vi "Save_Info.vi"(8 "error in (no error)":errorcluster, 11 "Class in":refnum<class "Installer.lvclass">) -> (0 "error out":errorcluster, 3 "Class out":refnum<class "Installer.lvclass">)   [LabVIEW 2020, in "Installer.lvclass"]
uses:
  <vilib>/AppBuilder/IB_Classes/Installer/Installer.lvclass
  <vilib>/AppBuilder/IB_RW_Project/IB_RW_Project_PropBag_Action.ctl
  <resource>/Framework/Providers/Builds/Installer/CDK_sTypeDef_StorageReadWrite.ctl
  <vilib>/AppBuilder/IB_RW_Project/IB_RW_Project_Installer_Data.ctl
  <resource>/Framework/Providers/Builds/Installer/CDK_sTypeDef_Languages.ctl
  <resource>/Framework/Providers/Builds/Installer/CDK_sTypeDef_ProductVersion.ctl
panel:
  in  "Installer":T1={"author"="", "productName"="", "buildSpecName"="", "hide"=FALSE, "requireLVDevSys"=FALSE, "autoIncrement"=FALSE, "includeError"=FALSE, "readmeID"="", "buildLocation"=path "", "mediaSize"=0, "language"=9, "productVersion"={"Major"=1, "Minor"=0, "Update"=0}, "defaultDir"="", "web service itemIDs"=[], "installerName"=""} {"productVersion"."Update" step=1; "productVersion"."Minor" step=1; "productVersion"."Major" step=1; "language" items=["English"=9, "German"=7, "French"=12, "Japanese"=17, "Korean"=18, "Chinese (Simplified)"=2052]}
  # "."
  # "."
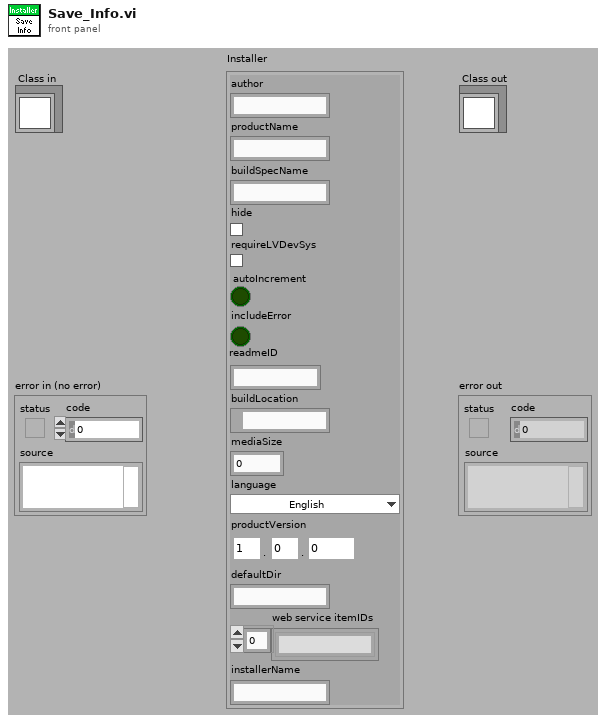
[diagram p1: front panel]
types:
  T1 = typedef "IB_RW_Project_Installer_Data.ctl" = cluster{"author":string, "productName":string, "buildSpecName":string, "hide":bool, "requireLVDevSys":bool, "autoIncrement":bool, "includeError":bool, "readmeID":string, "buildLocation":path, "mediaSize":u16, "language":T2, "productVersion":T3, "defaultDir":string, "web service itemIDs":string[], "installerName":string}
  T2 = typedef "CDK_sTypeDef_Languages.ctl" = u16
  T3 = typedef "CDK_sTypeDef_ProductVersion.ctl" = cluster{"Major":u8, "Minor":u8, "Update":u16}
  T4 = typedef "IB_RW_Project_PropBag_Action.ctl" = enum16{"read", "write", "clear", "readPrevious", "writePrevious", "clearPrevious"}
  T5 = typedef "CDK_sTypeDef_StorageReadWrite.ctl" = enum16{"Read", "Write", "Empty", "readPrevious"}
  T6 = typedef "ItemRef.ctl" = u64
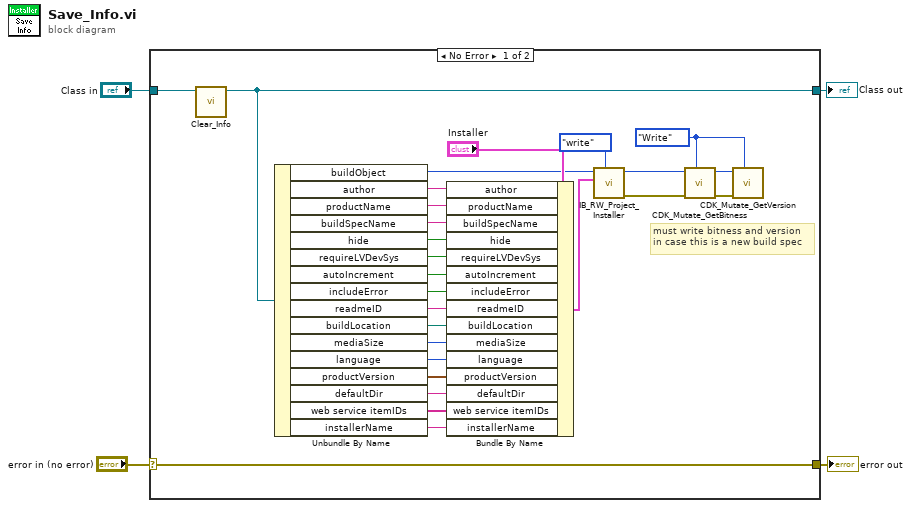
[diagram p0: block diagram]
diagram:
  n1 = case shown="No Error" "error in (no error)" {
    selector: "error in (no error)" -> [w29 w33]
    tunnel: [w29 w33] -> w3
    tunnel: [w13 w32] -> w1
    tunnel: "Class in" -> [w14 w32]
    frame No Error {
      w10 = CDK_sTypeDef_StorageReadWrite."Write" ("StorageAction")
      # "must write bitness and version\nin case this is a new build spec"
      n2 = call-dynamic "Clear_Info.vi"("Class in"=w14) -> ("Class out"=w13:refnum<class "Installer.lvclass">)  [unwired: 1 in, 9 out]
      n3 = Unbundle By Name(w13) -> ("buildObject"=w15:T6, "author"=w28:string, "productName"=w27:string, "buildSpecName"=w26:string, "hide"=w25:bool, "requireLVDevSys"=w24:bool, "autoIncrement"=w23:bool, "includeError"=w22:bool, "readmeID"=w21:string, "buildLocation"=w20:path, "mediaSize"=w19:u16, "language"=w18:T2, "productVersion"=w17:T3, "defaultDir"=w12:string, "web service itemIDs"=w6:string[], "installerName"=w5:string)
      n4 = Bundle By Name(cluster="Installer", "author"=w28, "productName"=w27, "buildSpecName"=w26, "hide"=w25, "requireLVDevSys"=w24, "autoIncrement"=w23, "includeError"=w22, "readmeID"=w21, "buildLocation"=w20, "mediaSize"=w19, "language"=w18, "productVersion"=w17, "defaultDir"=w12, "web service itemIDs"=w6, "installerName"=w5) -> (w30:T1)
      n5 = call <vilib>:"IB_RW_Project_Installer.vi"("action"=IB_RW_Project_PropBag_Action."write", "Installer in"=w30, "Object In"=w15) -> ("error out"=w8:errorcluster, "Object Out"=w9:T6)  [unwired: 2 in, 5 out]
      n6 = call <resource>:"CDK_Mutate_GetBitness.vi"("StorageAction"=w10, "ErrIn"=w8, "ObjectIn"=w9) -> ("ErrOut"=w7:errorcluster, "ObjectOut"=w11:T6)  [unwired: 7 out]
      n7 = call <resource>:"CDK_Mutate_GetVersion.vi"("StorageAction"=w10, "ErrIn"=w7, "ObjectIn"=w11) -> ()  [unwired: 6 in, 3 out]
    }
    frame Error {
    }
  }
  "error out" <- w3
  "Class out" <- w1
